vi "Labview lidar globals.vi"() -> ()   [LabVIEW 2017]
panel:
  out "Lidar VISA resource":refnum<visa-resource-name>
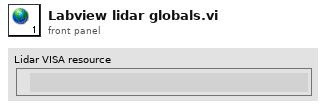
[diagram p1: front panel]
diagram:
